vi "Actor Core.vi"(8 "error in":errorcluster, 11 "Test Channel View in":refnum<class "Test Channel View.lvclass">) -> (0 "error out":errorcluster, 3 "Actor out":refnum<class "Actor.lvclass">)   [LabVIEW 2013, in "Test Channel View.lvlib" / "Test Channel View.lvclass"]
doc: "(<B>Filename</B>: Actor Framework.lvlib:Actor.lvclass:Actor Core.vi)\n\nReceives messages to the actor, reacts to them, and initiates any error handling that may shut the actor down.\n\nDescendant classes may override this VI to append parallel tasks for the actor to complete while it handles messages. Overrides use the Call Parent Method node."
uses:
  Test Channel View.lvclass
  <vilib>/ActorFramework/Actor/Actor.lvclass
  Resources/UI Controls/Tiles.ctl
  Resources/UI Controls/Tile.ctl
  Resources/UI Controls/Add Tile.ctl
  Resources/UI Controls/Delete Frame.ctl
  Test Channel View.lvclass/Test Channel View.ctl
  <vilib>/ActorFramework/Actor/Actor.lvclass/Actor.ctl
  <vilib>/ActorFrameworkMVC/View Actor/View Actor.lvclass
  <vilib>/ActorFramework/Message Enqueuer/Message Enqueuer.lvclass/Message Enqueuer.ctl
  Test Channel View Messages/Set Frame Visibility Msg/Set Frame Visibility Msg.lvclass/Set Frame Visibility Msg.ctl
  Test Channel View Messages/Update Tiles Msg/Update Tiles Msg.lvclass/Update Tiles Msg.ctl
  <vilib>/ActorFrameworkMVC/UI Controller Messages/Move Splitter Msg/Move Splitter Msg.lvclass/Move Splitter Msg.ctl
  <vilib>/Utility/miscctls.llb/LVPositionTypeDef.ctl
  <vilib>/ActorFrameworkMVC/UI Controller Messages/Move Subpanel Msg/Move Subpanel Msg.lvclass/Move Subpanel Msg.ctl
  <vilib>/ActorFrameworkMVC/UI Controller Messages/Insert Subpanel Msg/Insert Subpanel Msg.lvclass/Insert Subpanel Msg.ctl
  Models/Edit Test Channel Model Messages/Set Framed Test Channel Path Msg/Set Framed Test Channel Path Msg.lvclass/Set Framed Test Channel Path Msg.ctl
  Test Channel View Messages/Move Frame Msg/Move Frame Msg.lvclass/Move Frame Msg.ctl
  Models/Test Channel Model Messages/Set Framed Test Channel Path Msg/Set Framed Test Channel Path Msg.lvclass/Set Framed Test Channel Path Msg.ctl
  <vilib>/ActorFramework/Message Enqueuer/Init from Existing Queue.vi
  <vilib>/ActorFramework/Message Enqueuer/Enqueue.vi
  <vilib>/ActorFramework/Message Priority Queue/Priority Enqueue.vi
  <vilib>/ActorFramework/Message Enqueuer/Message Enqueuer.lvclass
  Test Channel View Messages/Set Frame Visibility Msg/Set Frame Visibility Msg.lvclass
  Test Channel View Messages/Update Tiles Msg/Update Tiles Msg.lvclass
  Test Channel View Messages/Move In Previous Page Msg/Move In Previous Page Msg.lvclass
  Test Channel View Messages/Move In Next Page Msg/Move In Next Page Msg.lvclass
  <vilib>/ActorFrameworkMVC/UI Controller Messages/Move Splitter Msg/Move Splitter Msg.lvclass
  <vilib>/ActorFrameworkMVC/UI Controller Messages/Move Subpanel Msg/Move Subpanel Msg.lvclass
  <vilib>/ActorFrameworkMVC/UI Controller Messages/Insert Subpanel Msg/Insert Subpanel Msg.lvclass
  Models/Test Node Model Messages/Preview Test Node Msg/Preview Test Node Msg.lvclass
  Models/Test Node Model Messages/Update Tiles Info Msg/Update Tiles Info Msg.lvclass
  Models/Test Node Model Messages/Update Previous Button Visibility Msg/Update Previous Button Visibility Msg.lvclass
  Models/Test Node Model Messages/Update Next Button Visibility Msg/Update Next Button Visibility Msg.lvclass
  Models/Create Test Channel Model Messages/Reinitialize All Msg/Reinitialize All Msg.lvclass
  Models/Create Test Channel Model Messages/Update Sensor Names Msg/Update Sensor Names Msg.lvclass
  Models/Create Test Channel Model Messages/Key Focus Msg/Key Focus Msg.lvclass
  Test Channel View Messages/Move Out Next Page Msg/Move Out Next Page Msg.lvclass
  Models/Test Channel Model Messages/Next Page Msg/Next Page Msg.lvclass
  Test Channel View Messages/Move Out Previous Page Msg/Move Out Previous Page Msg.lvclass
  Models/Test Channel Model Messages/Previous Page Msg/Previous Page Msg.lvclass
  Models/Edit Test Channel Model Messages/Set Framed Test Channel Path Msg/Set Framed Test Channel Path Msg.lvclass
  Models/Edit Test Channel Model Messages/Update Sensor Names Msg/Update Sensor Names Msg.lvclass
  Models/Edit Test Channel Model Messages/Initialize Edit Test Channel Msg/Initialize Edit Test Channel Msg.lvclass
  Test Channel View Messages/Move Frame Msg/Move Frame Msg.lvclass
  Models/Test Channel Model Messages/Set Framed Test Channel Path Msg/Set Framed Test Channel Path Msg.lvclass
  <vilib>/ActorFrameworkMVC/View Actor Messages/Get Model Enqueuer Msg/Get Model Enqueuer Msg.lvclass
  <vilib>/ActorFrameworkMVC/UI Controller Messages/Get Model Actor Enqueuer Msg/Get Model Actor Enqueuer Msg.lvclass
panel:
  in  "Frame":T1
  in  "Previous Button":bool
  in  "Next Button":bool
  in  "Add Tile":T2
  out "Tiles":T3
  in  "Back":bool
  # "测试通道"
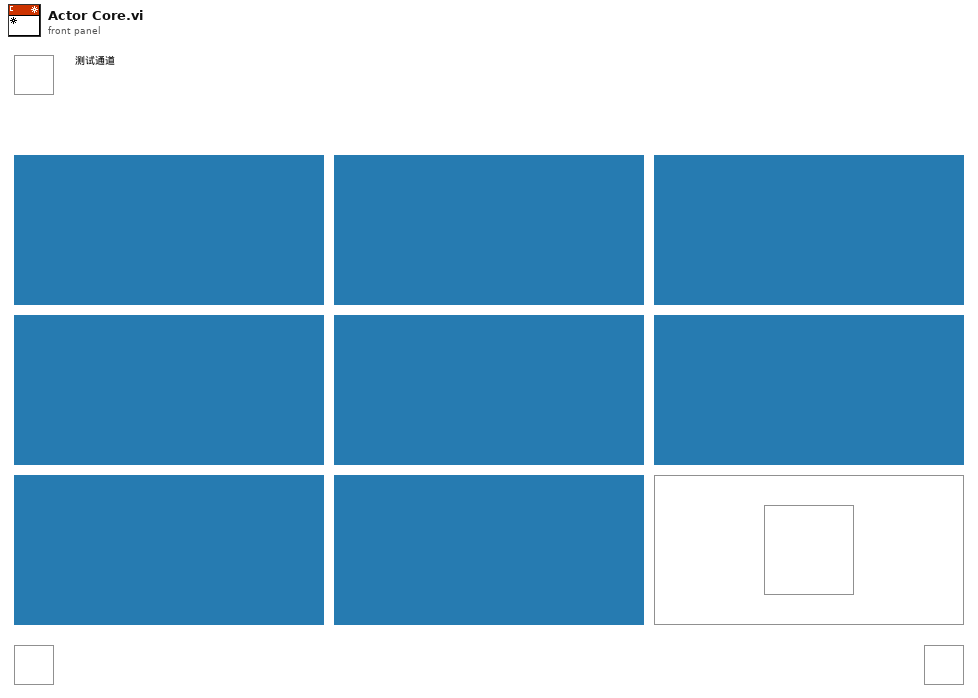
[diagram p1: front panel]
types:
  T1 = typedef "Delete Frame.ctl" = bool
  T2 = typedef "Add Tile.ctl" = bool
  T3 = typedef "Tiles.ctl" = cluster{"Tile 1":T4, "Tile 2":T4, "Tile 3":T4, "Tile 4":T4, "Tile 5":T4, "Tile 6":T4, "Tile 7":T4, "Tile 8":T4}
  T4 = typedef "Tile.ctl" = cluster{"Name":string, "Spec":string, "File Path":string}
  T5 = typedef "Test Channel View.lvlib/Test Channel View.lvclass/Events.ctl" = cluster{"Update Tiles Info":refnum<user-event>, "Set Previous Button Visibility":refnum<user-event>, "Set Next Button Visibility":refnum<user-event>, "Move In Previous":refnum<user-event>, "Move In Next":refnum<user-event>}
  T6 = typedef "LVPositionTypeDef.ctl" = cluster{"Left":i32, "Top":i32}
  T7 = enum8{"Enabled", "Disabled", "Disabled and Grayed Out"}
  T8 = typedef "Info Cluster.ctl" = cluster{"Name":string, "Spec":string, "File Path":string}
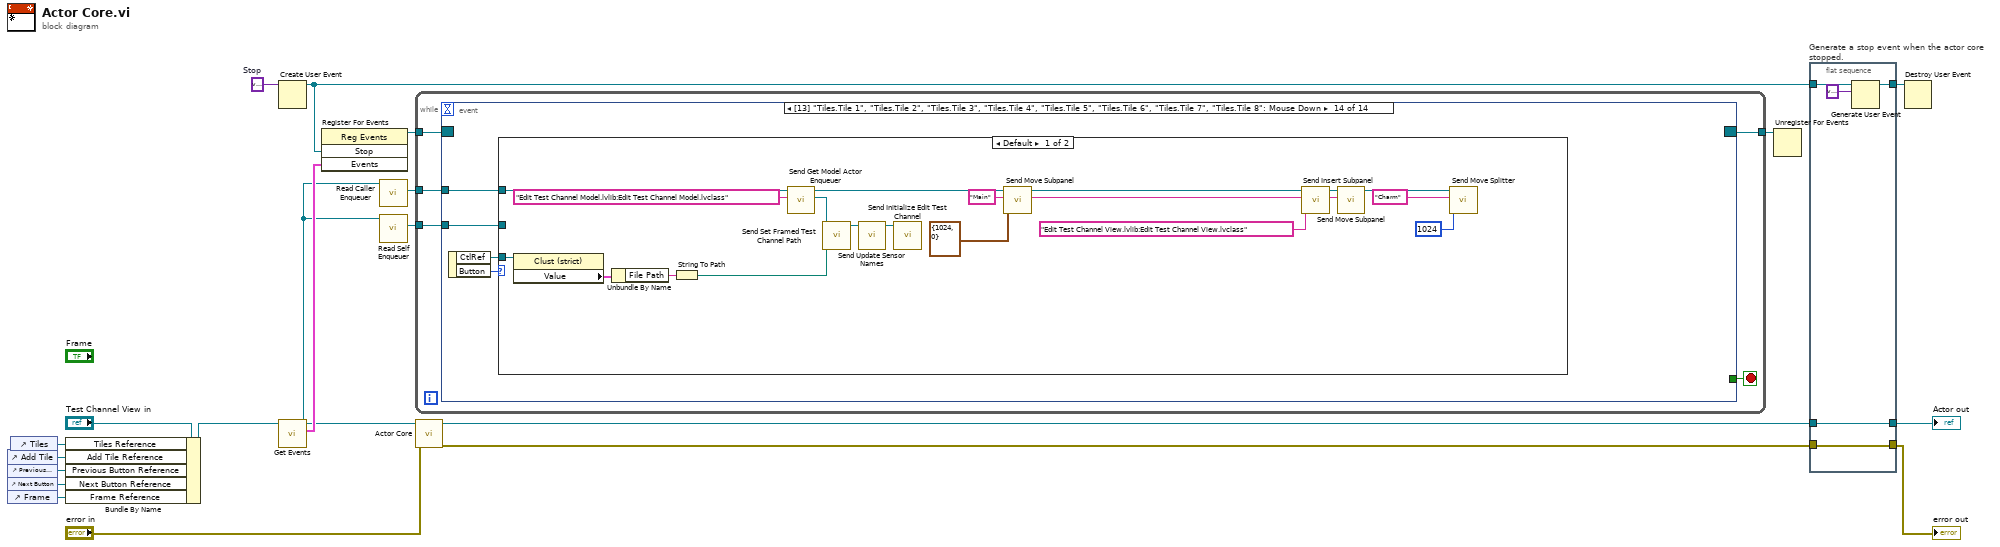
[diagram p0: block diagram]
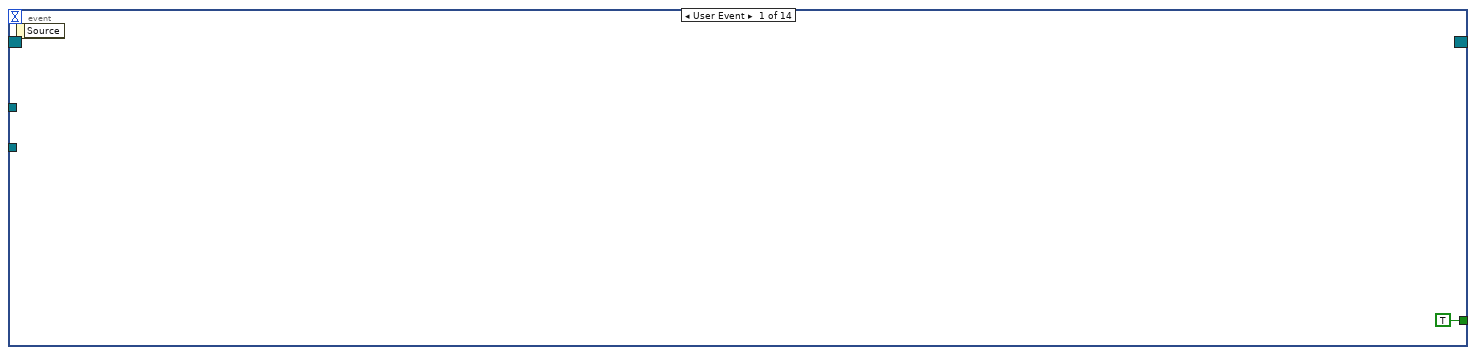
[diagram p2: hidden frame]
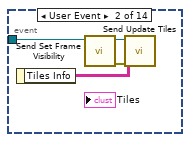
[diagram p3: hidden frame]
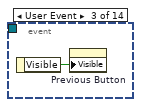
[diagram p4: hidden frame]
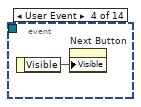
[diagram p5: hidden frame]
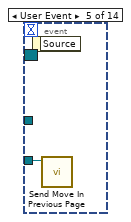
[diagram p6: hidden frame]
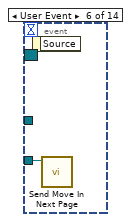
[diagram p7: hidden frame]
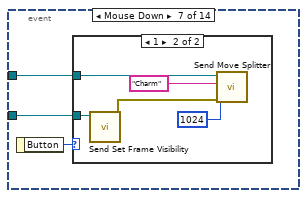
[diagram p8: hidden frame]
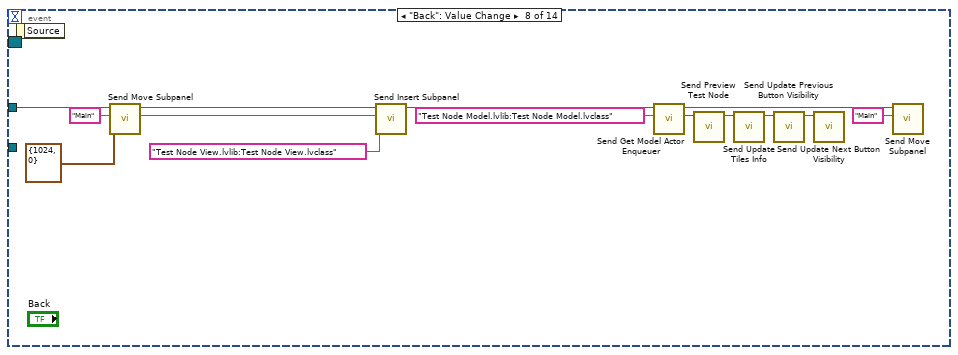
[diagram p10: hidden frame]
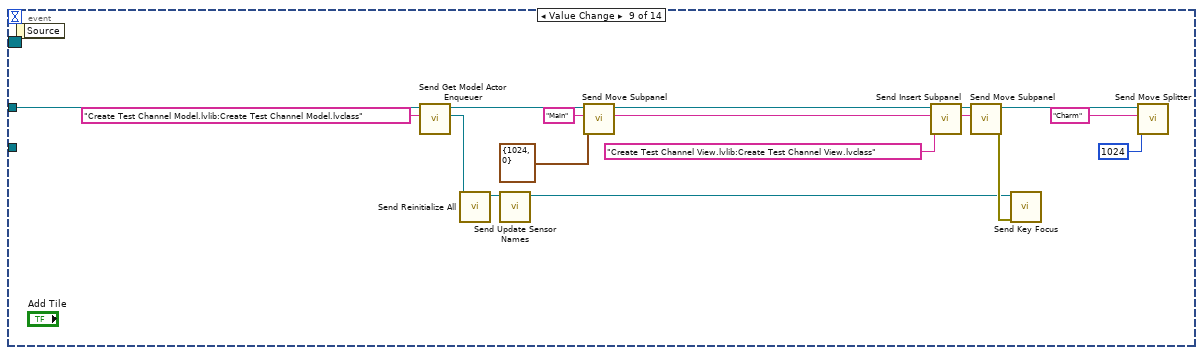
[diagram p11: hidden frame]
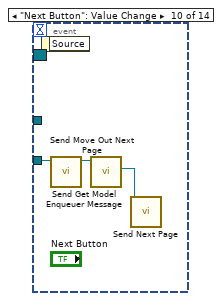
[diagram p12: hidden frame]
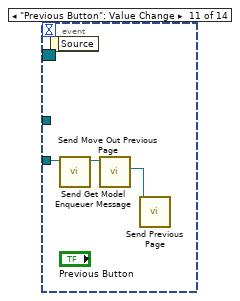
[diagram p13: hidden frame]
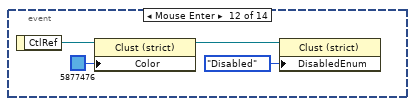
[diagram p14: hidden frame]
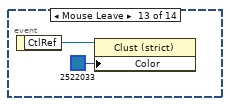
[diagram p15: hidden frame]
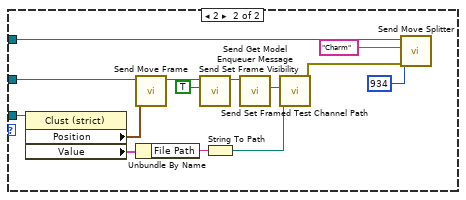
[diagram p16: hidden frame]
diagram:
  w21 = variant  # Stop
  n1 = control-ref of="Add Tile"() -> (w4:refnum<vi>)
  n2 = control-ref of="Previous Button"() -> (w5:refnum<vi>)
  n3 = control-ref of="Next Button"() -> (w6:refnum<vi>)
  n4 = control-ref of="Frame"() -> (w7:refnum<vi>)
  n5 = control-ref of="Tiles"() -> (w8:refnum<vi>)
  n6 = Bundle By Name(cluster="Test Channel View in", "Tiles Reference"=w8, "Add Tile Reference"=w4, "Previous Button Reference"=w5, "Next Button Reference"=w6, "Frame Reference"=w7) -> (w9:refnum<class "Test Channel View.lvclass">)
  n7 = Create User Event(user event datatype=w21) -> (user event=w12:refnum<user-event>)  [unwired: 1 in, 1 out]
  n8 = call "Get Events.vi"("Test Channel View in"=w9) -> ("Events"=w11:T5, "Test Channel View out"=w3:refnum<class "Test Channel View.lvclass">)  [unwired: 9 in]
  n9 = register-events(w12, w11) -> (reference out=w13:refnum<event-registration>)  [unwired: 2 in, 1 out]
  n10 = call <vilib>:"Read Caller Enqueuer.vi"("Actor"=w3) -> ("Caller Enqueuer"=w2:refnum<class "Message Enqueuer.lvclass">)  [unwired: 10 in]
  n11 = call <vilib>:"Read Self Enqueuer.vi"("Actor"=w3) -> ("Self Enqueuer"=w1:refnum<class "Message Enqueuer.lvclass">)  [unwired: 10 in]
  n12 = while {
    tunnel: [w26] -> w10
    tunnel: w13 -> [w24]
    tunnel: w2 -> [w23]
    tunnel: w1 -> [w22]
    stop <- w25 stop-if-true
    n13 = event shown="[13] \"Tiles.Tile 1\", \"Tiles.Tile 2\", \"Tiles.Tile 3\", \"Tiles.Tile 4\", \"Tiles.Tile 5\", \"Tiles.Tile 6\", \"Tiles.Tile 7\", \"Tiles.Tile 8\": Mouse Down" {
      selector: w24 -> [_ _ _ _ _ _ _ _ _ _ _ _ _ _]
      dyn-events: [_ _ _ _ _ _ _ _ _ _ _ _ _ _] -> w26
      timeout: _ -> [_ _ _ _ _ _ _ _ _ _ _ _ _ _]
      tunnel: [TRUE _ _ _ _ _ _ _ _ _ _ _ _ _] -> w25
      tunnel: w23 -> [_ _ _ _ _ _ w38 w44 w71 _ _ _ _ w84]
      tunnel: w22 -> [_ w31 _ _ w34 w35 w36 _ _ w73 w76 _ _ w85]
      event User Event {
        n14 = event-data() -> ()  [unwired: 1 in, 1 out]
      }
      event User Event {
        n15 = event-data() -> ("Tiles Info"=w29:string[][])  [unwired: 1 in]
        n16 = call "Send Set Frame Visibility.vi"("Message Enqueuer"=w31) -> ("error out"=w28:errorcluster, "Message Enqueuer out"=w30:refnum<class "Message Enqueuer.lvclass">)  [unwired: 9 in]
        n17 = call "Send Update Tiles.vi"("error in (no error)"=w28, "Channel Tiles Info"=w29, "Message Enqueuer"=w30) -> ()  [unwired: 7 in, 2 out]
      }
      event User Event {
        n18 = event-data() -> ("Visible"=w32:bool)  [unwired: 1 in]
        n19 = property on="Previous Button" class="Bool"("Visible"=w32) -> ()  [unwired: 2 in, 2 out]
      }
      event User Event {
        n20 = event-data() -> ("Visible"=w33:bool)  [unwired: 1 in]
        n21 = property on="Next Button" class="Bool"("Visible"=w33) -> ()  [unwired: 2 in, 2 out]
      }
      event User Event {
        n22 = event-data() -> ()  [unwired: 1 in, 1 out]
        n23 = call "Send Move In Previous Page.vi"("Message Enqueuer"=w34) -> ()  [unwired: 9 in, 2 out]
      }
      event User Event {
        n24 = event-data() -> ()  [unwired: 1 in, 1 out]
        n25 = call "Send Move In Next Page.vi"("Message Enqueuer"=w35) -> ()  [unwired: 9 in, 2 out]
      }
      event Mouse Down {
        n26 = event-data() -> ("Button"=w37:u16)  [unwired: 1 in]
        n27 = case shown="1" w37 {
          tunnel: w38 -> [_ w43]
          tunnel: w36 -> [_ w40]
          frame 0, Default {
          }
          frame 1 {
            n28 = call "Send Set Frame Visibility.vi"("Message Enqueuer"=w40) -> ("error out"=w39:errorcluster)  [unwired: 9 in, 1 out]
            n29 = call <vilib>:"Send Move Splitter.vi"("error in (no error)"=w39, "Splitter Position"=1024, "Splitter Name"="Charm", "Message Enqueuer"=w43) -> ()  [unwired: 6 in, 2 out]
          }
        }
      }
      event "Back": Value Change {
        w53 = "Main" ("Subpanel Name")
        n30 = event-data() -> ()  [unwired: 1 in, 1 out]
        n31 = call <vilib>:"Send Move Subpanel.vi"("Position (0,0)"=T6 {"Left"=1024, "Top"=0}, "Subpanel Name"=w53, "Message Enqueuer"=w44) -> ("Message Enqueuer out"=w56:refnum<class "Message Enqueuer.lvclass">)  [unwired: 7 in, 1 out]
        n32 = call <vilib>:"Send Insert Subpanel.vi"("View Name"="Test Node View.lvlib:Test Node View.lvclass" ("Subpanel Name"), "Subpanel Name"=w53, "Message Enqueuer"=w56) -> ("Message Enqueuer out"=w51:refnum<class "Message Enqueuer.lvclass">)  [unwired: 7 in, 1 out]
        n33 = call <vilib>:"Send Get Model Actor Enqueuer.vi"("Model Name"="Test Node Model.lvlib:Test Node Model.lvclass", "Message Enqueuer in"=w51) -> ("Reply"=w45:refnum<class "Message Enqueuer.lvclass">, "Message Enqueuer out"=w50:refnum<class "Message Enqueuer.lvclass">)  [unwired: 6 in, 2 out]
        n34 = call "Send Preview Test Node.vi"("Message Enqueuer"=w45) -> ("Message Enqueuer out"=w48:refnum<class "Message Enqueuer.lvclass">)  [unwired: 9 in, 1 out]
        n35 = call "Send Update Tiles Info.vi"("Message Enqueuer"=w48) -> ("Message Enqueuer out"=w47:refnum<class "Message Enqueuer.lvclass">)  [unwired: 9 in, 1 out]
        n36 = call "Send Update Previous Button Visibility.vi"("Message Enqueuer"=w47) -> ("Message Enqueuer out"=w46:refnum<class "Message Enqueuer.lvclass">)  [unwired: 9 in, 1 out]
        n37 = call "Send Update Next Button Visibility.vi"("Message Enqueuer"=w46) -> ()  [unwired: 9 in, 2 out]
        n38 = call <vilib>:"Send Move Subpanel.vi"("Subpanel Name"="Main", "Message Enqueuer"=w50) -> ()  [unwired: 8 in, 2 out]
      }
      event Value Change {
        w67 = "Main" ("Subpanel Name")
        n39 = event-data() -> ()  [unwired: 1 in, 1 out]
        n40 = call <vilib>:"Send Get Model Actor Enqueuer.vi"("Model Name"="Create Test Channel Model.lvlib:Create Test Channel Model.lvclass", "Message Enqueuer in"=w71) -> ("Reply"=w60:refnum<class "Message Enqueuer.lvclass">, "Message Enqueuer out"=w61:refnum<class "Message Enqueuer.lvclass">)  [unwired: 6 in, 2 out]
        n41 = call "Send Reinitialize All.vi"("Message Enqueuer"=w60) -> ("Message Enqueuer out"=w59:refnum<class "Message Enqueuer.lvclass">)  [unwired: 9 in, 1 out]
        n42 = call "Send Update Sensor Names.vi"("Message Enqueuer"=w59) -> ("Message Enqueuer out"=w57:refnum<class "Message Enqueuer.lvclass">)  [unwired: 9 in, 1 out]
        n43 = call <vilib>:"Send Move Subpanel.vi"("Position (0,0)"=T6 {"Left"=1024, "Top"=0}, "Subpanel Name"=w67, "Message Enqueuer"=w61) -> ("Message Enqueuer out"=w70:refnum<class "Message Enqueuer.lvclass">)  [unwired: 7 in, 1 out]
        n44 = call <vilib>:"Send Insert Subpanel.vi"("View Name"="Create Test Channel View.lvlib:Create Test Channel View.lvclass", "Subpanel Name"=w67, "Message Enqueuer"=w70) -> ("Message Enqueuer out"=w68:refnum<class "Message Enqueuer.lvclass">)  [unwired: 7 in, 1 out]
        n45 = call <vilib>:"Send Move Subpanel.vi"("Subpanel Name"=w67, "Message Enqueuer"=w68) -> ("error out"=w58:errorcluster, "Message Enqueuer out"=w66:refnum<class "Message Enqueuer.lvclass">)  [unwired: 8 in]
        n46 = call "Send Key Focus.vi"("error in (no error)"=w58, "Message Enqueuer"=w57) -> ()  [unwired: 8 in, 2 out]
        n47 = call <vilib>:"Send Move Splitter.vi"("Splitter Position"=1024, "Splitter Name"="Charm", "Message Enqueuer"=w66) -> ()  [unwired: 7 in, 2 out]
      }
      event "Next Button": Value Change {
        n48 = event-data() -> ()  [unwired: 1 in, 1 out]
        n49 = call "Send Move Out Next Page.vi"("Message Enqueuer"=w73) -> ("Message Enqueuer out"=w72:refnum<class "Message Enqueuer.lvclass">)  [unwired: 9 in, 1 out]
        n50 = call <vilib>:"Send Get Model Enqueuer Message.vi"("Message Enqueuer in"=w72) -> ("Reply"=w74:refnum<class "Message Enqueuer.lvclass">)  [unwired: 7 in, 3 out]
        n51 = call "Send Next Page.vi"("Message Enqueuer"=w74) -> ()  [unwired: 9 in, 2 out]
      }
      event "Previous Button": Value Change {
        n52 = event-data() -> ()  [unwired: 1 in, 1 out]
        n53 = call "Send Move Out Previous Page.vi"("Message Enqueuer"=w76) -> ("Message Enqueuer out"=w75:refnum<class "Message Enqueuer.lvclass">)  [unwired: 9 in, 1 out]
        n54 = call <vilib>:"Send Get Model Enqueuer Message.vi"("Message Enqueuer in"=w75) -> ("Reply"=w77:refnum<class "Message Enqueuer.lvclass">)  [unwired: 7 in, 3 out]
        n55 = call "Send Previous Page.vi"("Message Enqueuer"=w77) -> ()  [unwired: 9 in, 2 out]
      }
      event Mouse Enter {
        n56 = event-data() -> ("CtlRef"=w78:refnum<vi>)  [unwired: 1 in]
        n57 = property class="Clust (strict)"(reference=w78, "Color"=u32 5877476) -> (reference out=w80:refnum<vi>)  [unwired: 1 in, 1 out]
        n58 = property class="Clust (strict)"(reference=w80, "DisabledEnum"=T7."Disabled" ("Disabled")) -> ()  [unwired: 1 in, 2 out]
      }
      event Mouse Leave {
        n59 = event-data() -> ("CtlRef"=w82:refnum<vi>)  [unwired: 1 in]
        n60 = property class="Clust (strict)"(reference=w82, "Color"=u32 2522033) -> ()  [unwired: 1 in, 2 out]
      }
      event Mouse Down {
        n61 = event-data() -> ("CtlRef"=w87:refnum<vi>, "Button"=w86:u16)  [unwired: 1 in]
        n62 = case shown="Default" w86 {
          tunnel: w87 -> [w104 w119]
          tunnel: w85 -> [_ w118]
          tunnel: w84 -> [w105 w114]
          frame Default {
            w93 = "Main" ("Subpanel Name")
            n63 = property class="Clust (strict)"(reference=w104) -> ("Value"=w101:T4)  [unwired: 1 in, 2 out]
            n64 = Unbundle By Name(w101) -> ("File Path"=w100:string)
            n65 = String To Path(string=w100) -> (path=w99:path)
            n66 = call <vilib>:"Send Get Model Actor Enqueuer.vi"("Model Name"="Edit Test Channel Model.lvlib:Edit Test Channel Model.lvclass", "Message Enqueuer in"=w105) -> ("Reply"=w102:refnum<class "Message Enqueuer.lvclass">, "Message Enqueuer out"=w89:refnum<class "Message Enqueuer.lvclass">)  [unwired: 6 in, 2 out]
            n67 = call "Send Set Framed Test Channel Path.vi"("Framed Test Channel Path"=w99, "Message Enqueuer"=w102) -> ("Message Enqueuer out"=w98:refnum<class "Message Enqueuer.lvclass">)  [unwired: 8 in, 1 out]
            n68 = call "Send Update Sensor Names.vi"("Message Enqueuer"=w98) -> ("Message Enqueuer out"=w88:refnum<class "Message Enqueuer.lvclass">)  [unwired: 9 in, 1 out]
            n69 = call "Send Initialize Edit Test Channel.vi"("Message Enqueuer"=w88) -> ()  [unwired: 9 in, 2 out]
            n70 = call <vilib>:"Send Move Subpanel.vi"("Position (0,0)"=T6 {"Left"=1024, "Top"=0}, "Subpanel Name"=w93, "Message Enqueuer"=w89) -> ("Message Enqueuer out"=w90:refnum<class "Message Enqueuer.lvclass">)  [unwired: 7 in, 1 out]
            n71 = call <vilib>:"Send Insert Subpanel.vi"("View Name"="Edit Test Channel View.lvlib:Edit Test Channel View.lvclass", "Subpanel Name"=w93, "Message Enqueuer"=w90) -> ("Message Enqueuer out"=w92:refnum<class "Message Enqueuer.lvclass">)  [unwired: 7 in, 1 out]
            n72 = call <vilib>:"Send Move Subpanel.vi"("Subpanel Name"=w93, "Message Enqueuer"=w92) -> ("Message Enqueuer out"=w94:refnum<class "Message Enqueuer.lvclass">)  [unwired: 8 in, 1 out]
            n73 = call <vilib>:"Send Move Splitter.vi"("Splitter Position"=1024, "Splitter Name"="Charm", "Message Enqueuer"=w94) -> ()  [unwired: 7 in, 2 out]
          }
          frame 2 {
            n74 = property class="Clust (strict)"(reference=w119) -> ("Position"=w117:T6, "Value"=w110:T8)  [unwired: 1 in, 2 out]
            n75 = call "Send Move Frame.vi"("Position"=w117, "Message Enqueuer"=w118) -> ("Message Enqueuer out"=w116:refnum<class "Message Enqueuer.lvclass">)  [unwired: 8 in, 1 out]
            n76 = Unbundle By Name(w110) -> ("File Path"=w109:string)
            n77 = call "Send Set Frame Visibility.vi"("Visible (F)"=TRUE, "Message Enqueuer"=w116) -> ("Message Enqueuer out"=w111:refnum<class "Message Enqueuer.lvclass">)  [unwired: 8 in, 1 out]
            n78 = String To Path(string=w109) -> (path=w108:path)
            n79 = call <vilib>:"Send Get Model Enqueuer Message.vi"("Message Enqueuer in"=w111) -> ("Reply"=w106:refnum<class "Message Enqueuer.lvclass">)  [unwired: 7 in, 3 out]
            n80 = call "Send Set Framed Test Channel Path.vi"("Framed Test Channel Path"=w108, "Message Enqueuer"=w106) -> ("error out"=w107:errorcluster)  [unwired: 8 in, 1 out]
            n81 = call <vilib>:"Send Move Splitter.vi"("error in (no error)"=w107, "Splitter Position"=934, "Splitter Name"="Charm", "Message Enqueuer"=w114) -> ()  [unwired: 6 in, 2 out]
          }
        }
      }
    }
  }
  n82 = call-parent "Actor Core.vi"("error in"="error in", "View Actor in"=w3) -> ("error out"=w16:errorcluster, "Actor out"=w17:refnum<class "Actor.lvclass">)  [unwired: 8 in]
  n83 = Unregister For Events(event registration refnum=w10) -> ()  [unwired: 1 in, 1 out]
  n84 = flat-sequence "Generate a stop event when the actor core stopped." {
    tunnel: w12 -> [w124]
    tunnel: [w122] -> w20
    tunnel: w17 -> [w121]
    tunnel: w16 -> [w120]
    tunnel: [w121] -> w15
    tunnel: [w120] -> w14
    frame #0 {
      n85 = Generate User Event(user event=w124, event data cluster=variant ("event data")) -> (user event out=w122:refnum<user-event>)  [unwired: 2 in, 1 out]
    }
  }
  n86 = Destroy User Event(user event=w20) -> ()  [unwired: 1 in, 1 out]
  "error out" <- w14
  "Actor out" <- w15
